vi "2D Array Teil ersetzen.vi"(8 "Neues Element/Teil-Array":string[](array[string]), 9 "Spalte":i32, 10 "Zeile":i32, 11 "Eingangs Array":string[][](array[string])=[["", "", "", "", "", "", "", "", "", "1", "", "", "", "", "", "", "", "", "", "", "", "", "", "", "", "", "", "", "", ""], ["", "", "", "", "", "", "", "", "", "2", "", "", "", "", "", "", "", "", "", "", "", "", "", "", "", "", "", "", "", ""], ["", "", "", "", "", "", "", "", "", "3", "", "", "", "", "", "", "", "", "", "", "", "", "", "", "", "", "", "", "", ""], ["", "", "", "", "", "", "", "", "", "4", "", "", "", "", "", "", "", "", "", "", "", "", "", "", "", "", "", "", "", ""], ["", "", "", "", "", "", "", "", "", "5", "", "", "", "", "", "", "", "", "", "", "", "", "", "", "", "", "", "", "", ""], ["", "", "", "", "", "", "", "", "", "6", "", "", "", "", "", "", "", "", "", "", "", "", "", "", "", "", "", "", "", ""], ["", "", "", "", "", "", "", "", "", "7", "", "", "", "", "", "", "", "", "", "", "", "", "", "", "", "", "", "", "", ""], ["", "", "", "", "", "", "", "", "", "8", "", "", "", "", "", "", "", "", "", "", "", "", "", "", "", "", "", "", "", ""], ["", "", "", "", "", "", "", "", "", "9", "", "", "", "", "", "", "", "", "", "", "", "", "", "", "", "", "", "", "", ""], ["", "", "", "", "", "", "", "", "", "10", "", "", "", "", "", "", "", "", "", "", "", "", "", "", "", "", "", "", "", ""], ["", "", "", "", "", "", "", "", "", "", "", "", "", "", "", "", "", "", "", "", "", "", "", "", "", "", "", "", "", ""], ["", "", "", "", "", "", "", "", "", "", "", "", "", "", "", "", "", "", "", "", "", "", "", "", "", "", "", "", "", ""], ["", "", "", "", "", "", "", "", "", "", "", "", "", "", "", "", "", "", "", "", "", "", "", "", "", "", "", "", "", ""], ["", "", "", "", "", "", "", "", "", "", "", "", "", "", "", "", "", "", "", "", "", "", "", "", "", "", "", "", "", ""], ["", "", "", "", "", "", "", "", "", "", "", "", "", "", "", "", "", "", "", "", "", "", "", "", "", "", "", "", "", ""], ["", "", "", "", "", "", "", "", "", "", "", "", "", "", "", "", "", "", "", "", "", "", "", "", "", "", "", "", "", "0"]]) -> (3 "Ausgangs Array":string[][](array[string]))   [LabVIEW 2020, in "EPA 1065.lvlib" / "Gas Analyzer Drift 1065-550.lvlib"]
uses:
  Gas Analyzer Drift 1065-550.lvlib
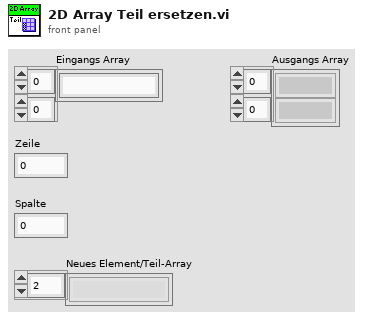
[diagram p1: front panel]
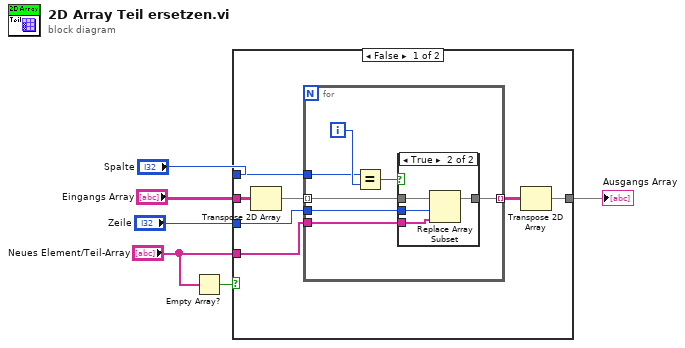
[diagram p0: block diagram]
diagram:
  n1 = Empty Array?(array="Neues Element/Teil-Array") -> (empty?=w1:bool)
  n2 = case shown="False" w1 {
    tunnel: "Spalte" -> [w13 _]
    tunnel: "Zeile" -> [w12 _]
    tunnel: [w9 w26] -> w4
    tunnel: "Eingangs Array" -> [w8 w26]
    tunnel: "Neues Element/Teil-Array" -> [w7 _]
    frame False {
      n3 = Transpose 2D Array(2D array=w8) -> (transposed array=w10:string[][])
      n4 = for {
        tunnel: w10 -> [w17] mode=indexing
        tunnel: w13 -> [w19]
        tunnel: w7 -> [w16]
        tunnel: w12 -> [w15]
        tunnel: [w14] -> w11 mode=indexing
        i -> [w20]
        n5 = Equal?(x=w19, y=w20) -> (x = y?=w18:bool)
        n6 = case shown="True" w18 {
          tunnel: w17 -> [w21 w25]
          tunnel: w16 -> [_ w24]
          tunnel: w15 -> [_ w23]
          tunnel: [w21 w22] -> w14
          frame False {
          }
          frame True {
            n7 = Replace Array Subset(array=w25, new element=w24, index=w23) -> (w22:string[])
          }
        }
      }
      n8 = Transpose 2D Array(2D array=w11) -> (transposed array=w9:string[][])
    }
    frame True {
    }
  }
  "Ausgangs Array" <- w4
